vi "Write Server Internal UEs.vi"(8 "error in (no error)":errorcluster, 10 "Server Internal UEs":T1, 11 "SignalGeneratorService in":refnum<class "Random_Data.lvclass">) -> (0 "error out":errorcluster, 3 "SignalGeneratorService out":refnum<class "Random_Data.lvclass">)   [LabVIEW 2021, in "Stream_server.lvlib" / "Random_Data.lvclass"]
uses:
  Random_Data.lvclass
  typeDefs/Server Internal UEs.ctl
  typeDefs/Server Internal Message.ctl
  Random_Data.lvclass/Random_Data.ctl
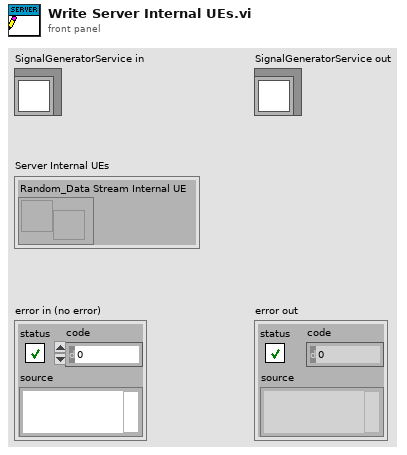
[diagram p1: front panel]
types:
  T1 = typedef "Stream_server.lvlib/Random_Data.lvclass/Server Internal UEs.ctl" = cluster{"Random_Data Stream Internal UE":refnum<user-event>}
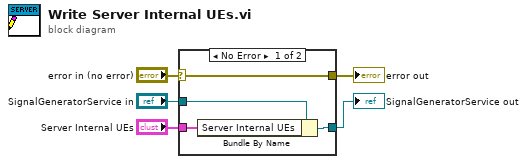
[diagram p0: block diagram]
diagram:
  n1 = case shown="No Error" "error in (no error)" {
    selector: "error in (no error)" -> [w9 w10]
    tunnel: [w9 w10] -> w4
    tunnel: [w7 w11] -> w2
    tunnel: "SignalGeneratorService in" -> [w8 w11]
    tunnel: "Server Internal UEs" -> [w6 _]
    frame No Error {
      n2 = Bundle By Name(cluster=w8, "Server Internal UEs"=w6) -> (w7:refnum<class "Random_Data.lvclass">)
    }
    frame Error {
    }
  }
  "error out" <- w4
  "SignalGeneratorService out" <- w2
